vi "Detect Pci Delay Generators.vi"(8 "error in (no error)":errorcluster) -> (0 "error out":errorcluster, 2 "Number of Generators":i32, 3 "Error":i32)   [LabVIEW 2009, in "POLARIS BME DG.lvlib"]
doc: "long DetectPciDelayGenerators(long* p_Error);"
uses:
  POLARIS BME DG.lvlib
  BME DLL/DelayGenerator.dll
panel:
  # "NOTICE -- YOU MUST LEAVE THIS NOTICE IN PLACE.  PER THE TERMS OF THE LICENSE BELOW, YOU MAY SUBLICENSE THIS SOFTWARE \nIN ANY WAY THAT DOES NOT CONFLICT WITH THIS LICENSE.\n\n### BSD License (http://www.opensource.org/licenses/bsd-license.php) Begin ###\n \nCopyright (c) 2011, Applied Energetics, http://www.appliedenergetics.com,\n                               Richard Schwerdtfeger, <rschwerdtfeger@appliedenergetics.com>\n\nAll rights reserved.\n\nRedistribution and use in source and binary forms, with or without modification, are permitted provided that the \nfollowing conditions are met:\n\n    * Redistributions of source code must retain the above copyright notice, this list of conditions and the following disclaimer.\n    * Redistributions in binary form must reproduce the above copyright notice, this list of conditions and the following disclaimer \n       in the documentation and/or other materials provided with the distribution.\n    * Neither the name of Richard Schwerdtfeger, Applied Energetics, Inc., nor the names of its contributors may be used to \n       endorse or promote products derived from this software without specific prior written permission.\n\nTHIS SOFTWARE IS PROVIDED BY THE COPYRIGHT HOLDERS AND CONTRIBUTORS \"AS IS\" AND ANY EXPRESS OR IMPLIED WARRANTIES, \nINCLUDING, BUT NOT LIMITED TO, THE IMPLIED WARRANTIES OF MERCHANTABILITY AND FITNESS FOR A PARTICULAR PURPOSE ARE \nDISCLAIMED. IN NO EVENT SHALL THE COPYRIGHT OWNER OR CONTRIBUTORS BE LIABLE FOR ANY DIRECT, INDIRECT, INCIDENTAL,\n SPECIAL, EXEMPLARY, OR CONSEQUENTIAL DAMAGES (INCLUDING, BUT NOT LIMITED TO, PROCUREMENT OF SUBSTITUTE GOODS OR \nSERVICES; LOSS OF USE, DATA, OR PROFITS; OR BUSINESS INTERRUPTION) HOWEVER CAUSED AND ON ANY THEORY OF LIABILITY, \nWHETHER IN CONTRACT, STRICT LIABILITY, OR TORT (INCLUDING NEGLIGENCE OR OTHERWISE) ARISING IN ANY WAY OUT OF THE USE \nOF THIS SOFTWARE, EVEN IF ADVISED OF THE POSSIBILITY OF SUCH DAMAGE.\n\n### BSD License End ###"
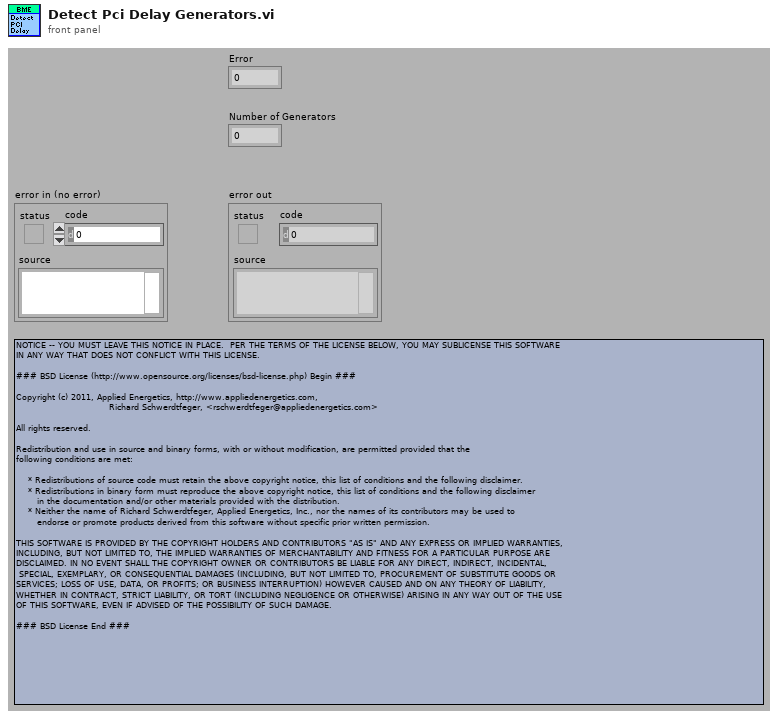
[diagram p1: front panel]
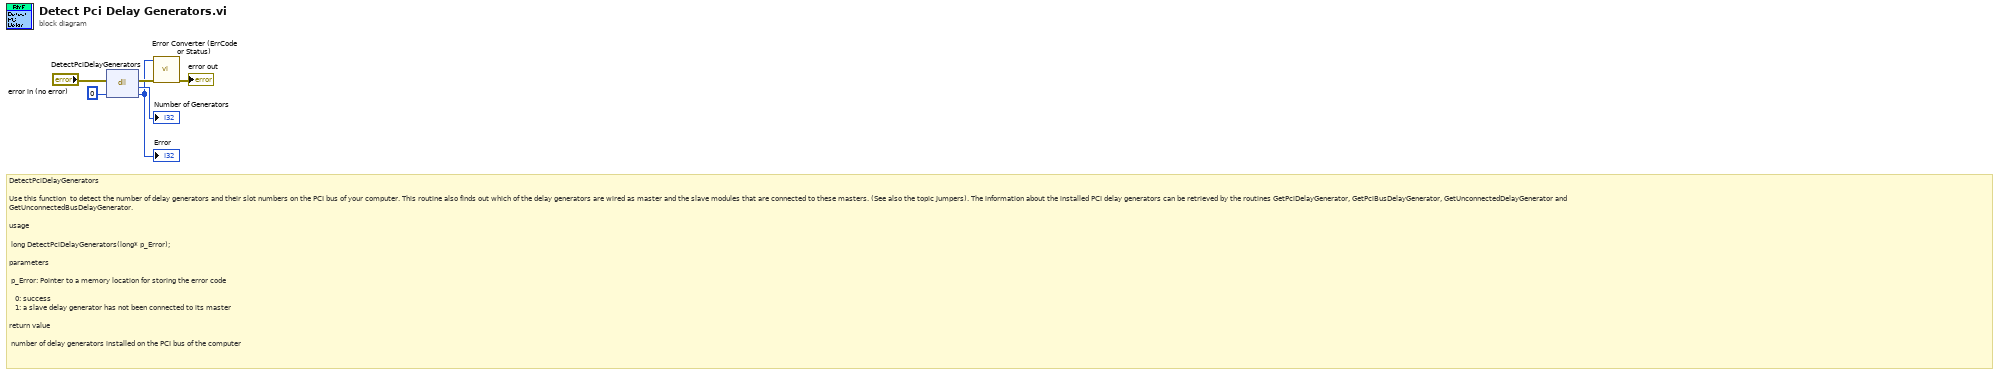
[diagram p0: block diagram]
diagram:
  # "DetectPciDelayGenerators\n\nUse this function  to detect the number of delay generators and their slot numbers on the PCI bus of your computer. This routine also finds out which of the delay generators are wired as master and the slave modules that are connected to these masters. (See also the topic Jumpers). The information about the installed PCI delay generators can be retrieved by the routines GetPciDelayGenerator, GetPciBusDelayGenerator, GetUnconnectedDelayGenerator and GetUnconnectedBusDelayGenerator.\n\nusage\n\n\tlong DetectPciDelayGenerators(long* p_Error);\n\nparameters\n\n\tp_Error:\tPointer to a memory location for storing the error code\n\n\t\t\t0:\tsuccess\n\t\t\t1:\ta slave delay generator has not been connected to its master\n\nreturn value\n\n\tnumber of delay generators installed on the PCI bus of the computer"
  n1 = dll-call lib="C:/CS Framework/LVSCC/LV2009/GPL/Projects/cs-framework/CSClass/CSPOLARIS/POLARIS BME DG/BME DLL/DelayGenerator.*" fn="DetectPciDelayGenerators"(error in="error in (no error)", "p_Error"=0) -> (error out=w3:errorcluster, →"Number of Generators":i32, "p_Error"=w1:i32)  [unwired: 2 in, 1 out]
  "Error" <- w1
  n2 = call "Error Converter (ErrCode or Status).vi"("error in (no error)"=w3, "error code"=w1) -> ("error out"=→"error out":errorcluster)  [unwired: 9 out]
